vi "turn relay off.vi"(8 "error in (no error)":errorcluster, 9 "on/off":bool, 10 "index":i32, 11 "hardware in":refnum<class "hardware.lvclass">) -> (0 "error out":errorcluster, 3 "hardware out":refnum<class "hardware.lvclass">)   [LabVIEW 2025, in "hardware.lvclass"]
uses:
  hardware.lvclass
  hardware.lvclass/hardware.ctl
  <vilib>/DAQmx/write.llb/DAQmx Write (Digital 1D Bool 1Chan 1Samp).vi
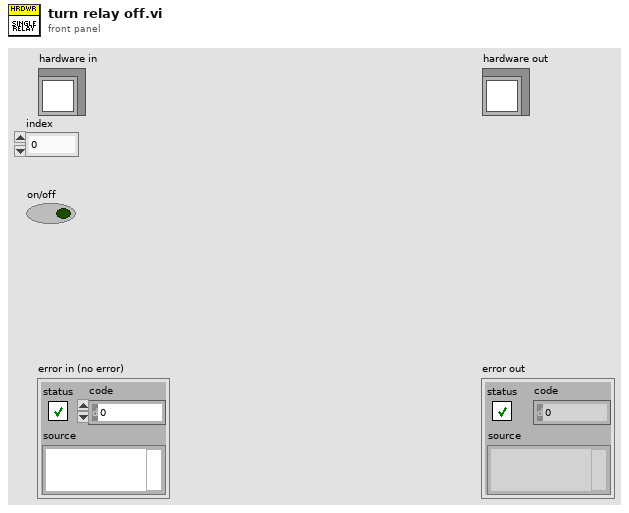
[diagram p1: front panel]
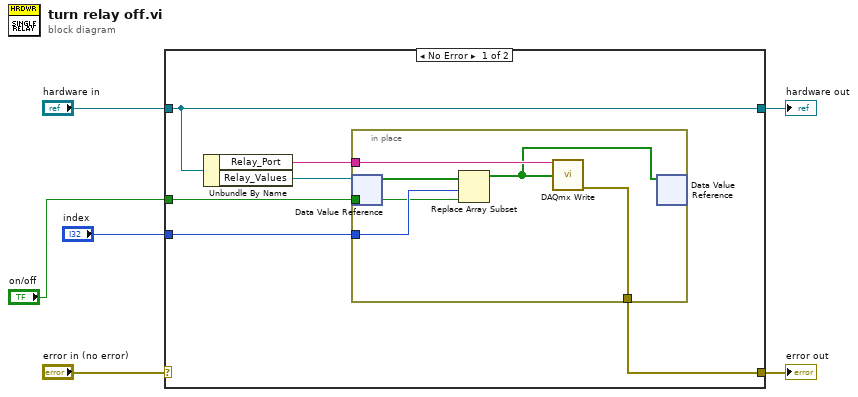
[diagram p0: block diagram]
diagram:
  n1 = case shown="No Error" "error in (no error)" {
    selector: "error in (no error)" -> [_ w19]
    tunnel: [w12 w20] -> w4
    tunnel: "hardware in" -> [w12 w20]
    tunnel: "index" -> [w9 _]
    tunnel: [w8 w19] -> w2
    tunnel: "on/off" -> [w7 _]
    frame No Error {
      n2 = Unbundle By Name(w12) -> ("Relay_Port"=w10:string, "Relay_Values"=w11:refnum<data-value>)
      n3 = in-place {
        in-place-border: w10 -> [w16]
        in-place-border: w9 -> [w17]
        in-place-border: [w14] -> w8
        in-place-border: w7 -> [w13]
        n4 = in-place-dvr #1(w11) -> (w18:bool[])  [unwired: 1 out]
        n5 = Replace Array Subset(array=w18, new element=w13, index=w17) -> (w15:bool[])
        n6 = call-poly <vilib>:"DAQmx Write.vi"("task/channels in"=w16, "data"=w15) -> ("error out"=w14:errorcluster)  [unwired: 11 in, 2 out]
        n7 = in-place-dvr #1(w15) -> ()  [unwired: 2 out]
      }
    }
    frame Error {
    }
  }
  "error out" <- w2
  "hardware out" <- w4
